vi "Read Subdiagrams.vi"(8 "error in (no error)":errorcluster, 11 "Structure in":refnum<class "Structure.lvclass">) -> (0 "error out":errorcluster, 2 "Subdiagrams":map{string, T1}(c390), 3 "Structure out":refnum<class "Structure.lvclass">)   [LabVIEW 2025, in "Structure.lvclass"]
uses:
  Structure.lvclass
  Controls/Subdiagram.ctl
  Structure.lvclass/Structure.ctl
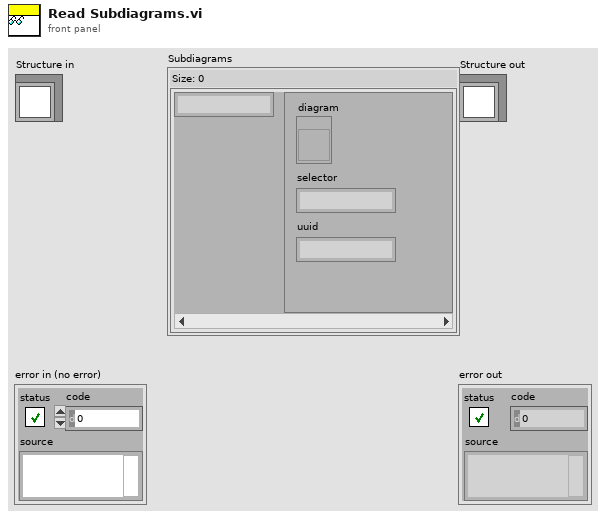
[diagram p1: front panel]
types:
  T1 = typedef "Subdiagram.ctl" = cluster{"diagram":refnum<vi>, "selector":string, "uuid":string}
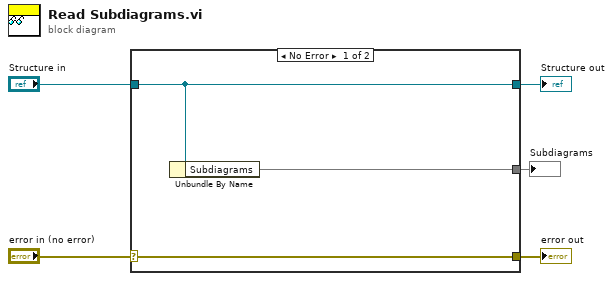
[diagram p0: block diagram]
diagram:
  n1 = case shown="No Error" "error in (no error)" {
    selector: "error in (no error)" -> [w8 w9]
    tunnel: [w8 w9] -> w4
    tunnel: [w7 w10] -> w2
    tunnel: "Structure in" -> [w7 w10]
    tunnel: [w6 _] -> w1
    frame No Error {
      n2 = Unbundle By Name(w7) -> ("Subdiagrams"=w6:map{string, T1})
    }
    frame Error {
    }
  }
  "error out" <- w4
  "Structure out" <- w2
  "Subdiagrams" <- w1
